vi "Connect.vi"(8 "error in (no error)":errorcluster, 11 "FunctionGenerator in":refnum<class "FunctionGenerator.lvclass">) -> (0 "error out":errorcluster, 3 "FunctionGenerator out":refnum<class "FunctionGenerator.lvclass">)   [LabVIEW 2019, in "FunctionGenerator.lvlib" / "FunctionGenerator.lvclass"]
uses:
  Library/FunctionGenerator.lvclass
  builds/Instruments/Instruments.lvlibp/Library/Instruments.lvclass
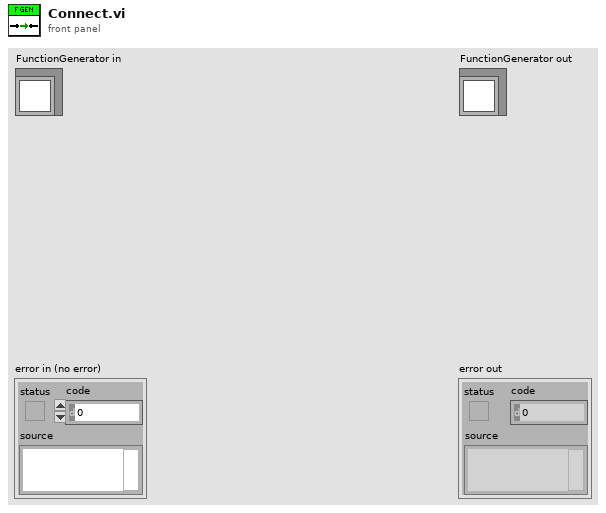
[diagram p1: front panel]
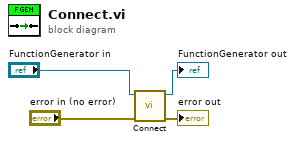
[diagram p0: block diagram]
diagram:
  n1 = call-parent "Connect.vi"("error in (no error)"="error in (no error)", "Instruments in"="FunctionGenerator in") -> ("error out"=→"error out":errorcluster, "Instruments out"=→"FunctionGenerator out":refnum<class "FunctionGenerator.lvclass">)  [unwired: 8 in]
